vi "多列列表框根据窗格缩放.vi"(8 "error in (no error)":errorcluster caption="错误输入（无错误）") -> (0 "error out":errorcluster caption="错误输出")   [LabVIEW 2020]
uses:
  <vilib>/Utility/miscctls.llb/LVRowAndColumnTypeDef.ctl
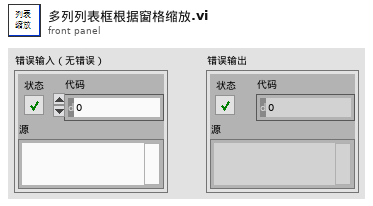
[diagram p1: front panel]
types:
  T1 = typedef "LVRowAndColumnTypeDef.ctl" = cluster{"Row":i32, "Column":i32}
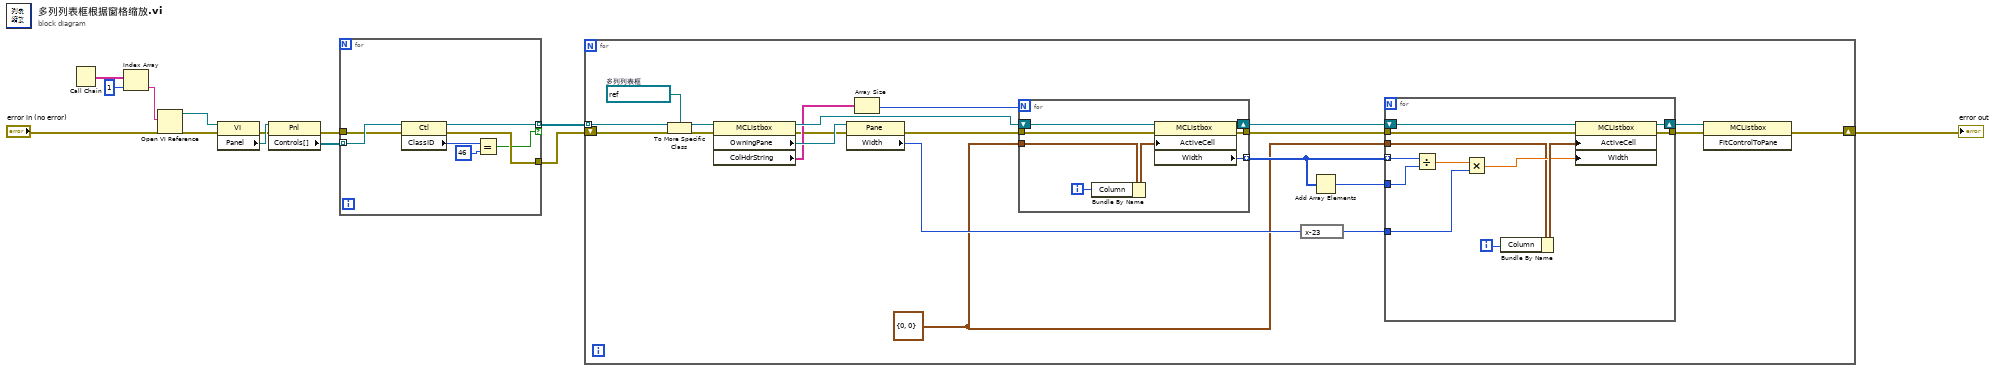
[diagram p0: block diagram]
diagram:
  n1 = Call Chain() -> (call chain=w13:string[])
  n2 = Index Array(array=w13, index=1 ("索引")) -> (element=w11:string)
  n3 = Open VI Reference(vi path=w11, error in (no error)="error in (no error)") -> (vi reference=w10:refnum<vi>, error out=w5:errorcluster)  [unwired: 4 in]
  n4 = property class="VI"(reference=w10, error in=w5) -> (error out=w4:errorcluster, "Panel"=w9:refnum<vi>)  [unwired: 1 out]
  n5 = property class="Pnl"(reference=w9, error in=w4) -> (error out=w3:errorcluster, "Controls[]"=w8:refnum<vi>[])  [unwired: 1 out]
  n6 = for {
    tunnel: w8 -> [w20] mode=indexing
    tunnel: [w17] -> w7 mode=indexing if=w14
    tunnel: w3 -> [w16]
    tunnel: [w15] -> w2
    n7 = property class="Ctl"(reference=w20, error in=w16) -> (reference out=w17:refnum<vi>, error out=w15:errorcluster, "ClassID"=w19:u32)
    n8 = Equal?(x=w19, y=u32 46) -> (x = y?=w14:bool)
  }
  n9 = for {
    tunnel: w7 -> [w33] mode=indexing
    shift-right: [w21] -> w1
    shift-left: w2 -> [w29]
    w30 = T1 {"Row"=0, "Column"=0} ("活动单元格:活动单元格")
    w32 = refnum<vi> refnum  # 多列列表框
    n10 = To More Specific Class(target class=w32, reference=w33, error in=w29) -> (specific class reference=w31:refnum<vi>, error out=w28:errorcluster)
    n11 = property class="MCListbox"(reference=w31, error in=w28) -> (reference out=w41:refnum<vi>, error out=w27:errorcluster, "OwningPane"=w40:refnum<vi>, "ColHdrString"=w35:string[])
    n12 = property class="Pane"(reference=w40, error in=w27) -> (error out=w26:errorcluster, "Width"=w36:u32)  [unwired: 1 out]
    n13 = Array Size(array=w35) -> (size(s)=w34:i32)
    n14 = for {
      N: w34 -> [_]
      tunnel: [w58] -> w37 mode=indexing
      tunnel: w30 -> [w56]
      tunnel: w26 -> [w55]
      tunnel: [w54] -> w25
      shift-right: [w57] -> w39
      shift-left: w41 -> [w61]
      i -> [w59]
      n15 = Bundle By Name(cluster=w56, "Column"=w59) -> (w60:T1)
      n16 = property class="MCListbox"(reference=w61, error in=w55, "ActiveCell"=w60) -> (reference out=w57:refnum<vi>, error out=w54:errorcluster, "Width"=w58:u32)
    }
    n17 = expression code="x-23"(w36) -> (w24:u32)
    n18 = Add Array Elements(numeric array=w37) -> (sum=w38:u32)
    n19 = for {
      tunnel: w37 -> [w53] mode=indexing
      tunnel: w38 -> [w52]
      tunnel: w30 -> [w47]
      tunnel: w25 -> [w46]
      tunnel: [w45] -> w22
      tunnel: w24 -> [w43]
      shift-right: [w42] -> w23
      shift-left: w39 -> [w51]
      i -> [w50]
      n20 = Divide(x=w53, y=w52) -> (x/y=w44:dbl)
      n21 = Multiply(x=w44, y=w43) -> (x*y=w48:dbl)
      n22 = Bundle By Name(cluster=w47, "Column"=w50) -> (w49:T1)
      n23 = property class="MCListbox"(reference=w51, error in=w46, "ActiveCell"=w49, "Width"=w48) -> (reference out=w42:refnum<vi>, error out=w45:errorcluster)
    }
    n24 = invoke class="MCListbox" method="FitControlToPane"(reference=w23, error in=w22) -> (error out=w21:errorcluster)  [unwired: 1 in, 2 out]
  }
  "error out" <- w1
